vi "finalProject_interfaceLabVIEW.vi"(5 "stop":bool) -> (1 "Últimos Valores Registados:":string[](array[string]), 2 "Array":string[](array[string]), 3 "Waveform Chart":dynamicdata(graph)=[{"t0"=timestamp(3816698513.7637887 s since 1904-01-01), "dt"=1.0, "Y"=[0.0]}, {"t0"=timestamp(3816698513.7637887 s since 1904-01-01), "dt"=1.0, "Y"=[28.961962479327045]}])   [LabVIEW 2024]
uses:
  <vilib>/Instr/_visa.llb/VISA Flush IO Buffer Mask.ctl
  <vilib>/Platform/TimedLoop/XDataNode/timing_clust.ctl
  <vilib>/Platform/TimedLoop/XDataNode/nitl_modes.ctl
  <vilib>/Platform/TimedLoop/XDataNode/wakeup.ctl
  <vilib>/Utility/file.llb/Write Delimited Spreadsheet (string).vi
  <vilib>/Instr/_visa.llb/VISA Configure Serial Port (Instr).vi
  <vilib>/platform/TimedLoop/XDataNode/XDataNode.xnode
  <vilib>/Platform/TimedLoop/XDataNode/XDNodeRunTimeDep.lvlib
panel:
  out "Luminosidade (%)":sgl(slide) scale=0.0..100.0
  out "Histórico de Valores:":string[][](table)
  out "State":bool
  in  "Porta de Comunicação":refnum<visa-resource-name>="COM3-1"
  in  "Temp Setpoint (ºC)":sgl(knob)=25.0 scale=15.0..30.0 scale format="%#_2f"
  out "Temp Medida (ºC)":dbl(slide) scale=10.0..30.0
  out "Última Mensagem recebida do Arduino:":string
  in  "Diretoria de Dados Guardados:":path=path "C:/Users/celin/Documents/Alexandre Escola/Universidade/FEUP - Faculdade de Engenharia do Porto/1º Semestre/ASM - Aplicações de Sistemas Mecatrónicos/Arduino+LabView/Results.xls"
  # "Verde: Sistema Operacional\nAmarelo: Sistema Não Operacional"
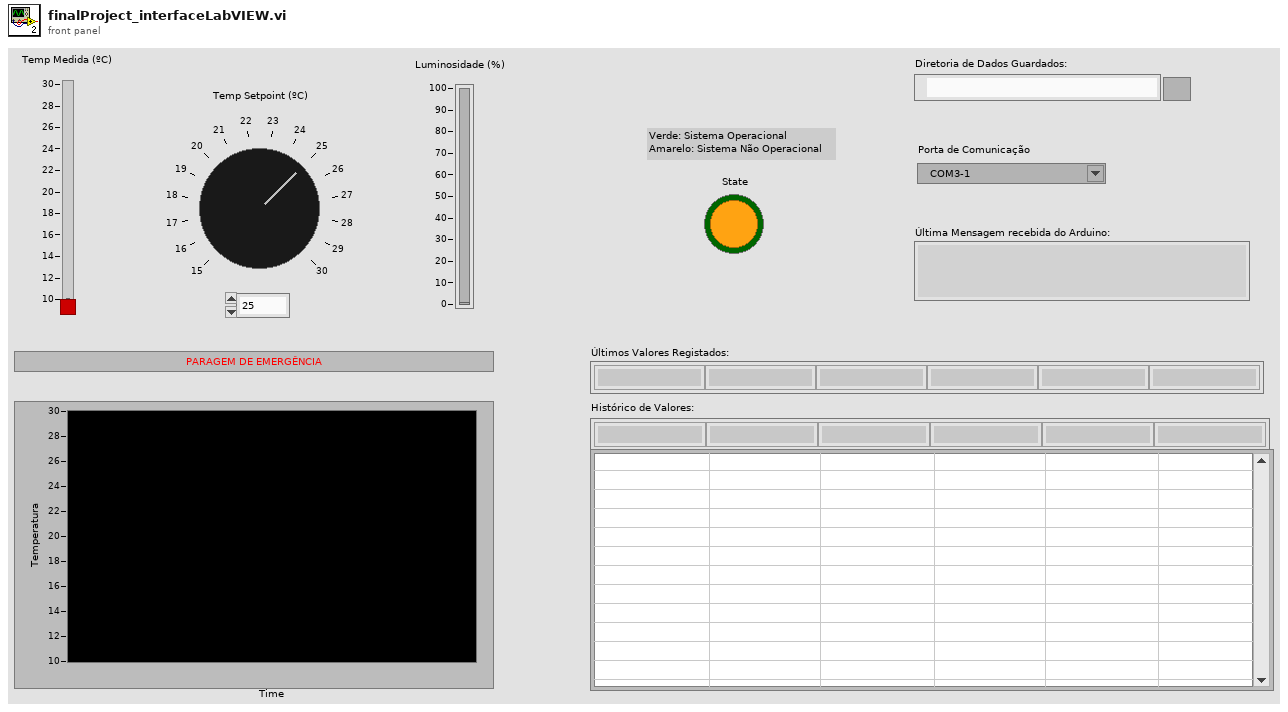
[diagram p1: front panel]
types:
  T1 = typedef "XDNodeRunTimeDep.lvlib/timing_clust.ctl" = cluster{"Expected End [f-1]":u64, "Actual End [f-1]":u64, "Finished Late? [f-1]":bool, "Expected End [i-1]":u64, "Actual End [i-1]":u64, "Finished Late? [i-1]":bool, "Expected Start [i]":u64, "Actual Start [i]":u64, "Expected Start [f]":u64, "Actual Start [f]":u64, "Source Name":string, "Structure Name":string, "Period":i64, "Deadline":i64, "Offset":i64, "Start":i64, "Priority":i32, "Timeout":i32, "Mode":T2, "Wakeup Reason":T3, "Error":errorcluster, "Source Type":string, "Secondary Source Type":string, "Global End Time":u64, "Global Start Time":u64, "Frame Duration":u64, "Iteration Duration":u64, "Assigned CPU":i32, "I/O Scan Engine Mode":u32}
  T2 = typedef "XDNodeRunTimeDep.lvlib/nitl_modes.ctl" = enum32{"No Change", "Process missed periods, maintain original phase", "Discard missed periods, maintain original phase", "Process missed periods, ignore original phase", "Discard missed periods, ignore original phase"}
  T3 = typedef "XDNodeRunTimeDep.lvlib/wakeup.ctl" = enum32{"Normal", "Aborted", "Asynchronous wakeup", "Timing source error", "Timed loop error", "Timeout"}
  T4 = typedef "VISA Flush IO Buffer Mask.ctl" = u16
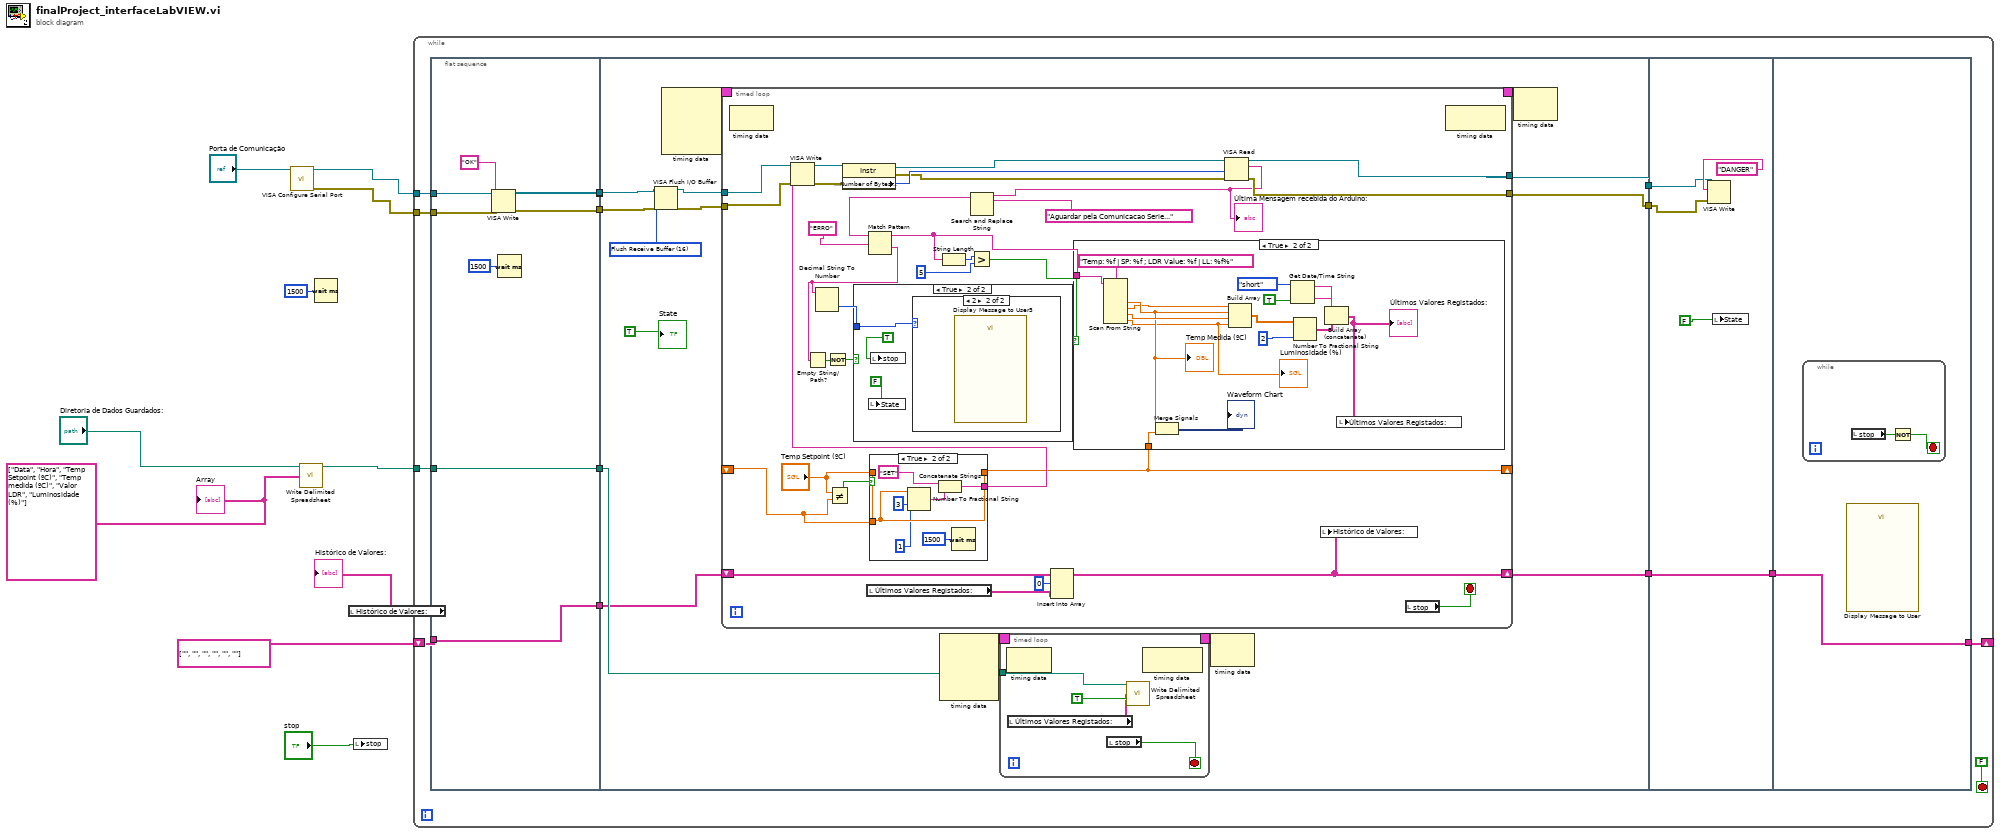
[diagram p0: block diagram]
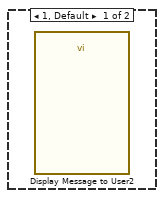
[diagram p3: hidden frame]
diagram:
  w8 = string[] ["Data", "Hora", "Temp Setpoint (ºC)", "Temp medida (ºC)", "Valor LDR", "Luminosidade (%)"]
  n1 = call-poly "VISA Configure Serial Port"("VISA resource name"="Porta de Comunicação") -> ("VISA resource name out"=w4:refnum<visa-resource-name>, "error out"=w5:errorcluster)  [unwired: 13 in]
  n2 = call-poly <vilib>:"Write Delimited Spreadsheet.vi"("file path (dialog if empty)"="Diretoria de Dados Guardados:", "1D data"=w8) -> ("new file path (Not A Path if cancelled)"=w7:path)  [unwired: 12 in, 1 out]
  n3 = Wait (ms)(milliseconds to wait=u32 1500) -> ()  [unwired: 1 out]
  n4 = local read "Histórico de Valores:"() -> (→"Histórico de Valores:":string[][])
  n5 = local write "stop"("stop") -> ()
  n6 = while {
    tunnel: w7 -> [w19]
    tunnel: w5 -> [w16]
    tunnel: w4 -> [w15]
    shift-right: [w12] -> _
    shift-left: string[][] [["", "", "", "", "", ""]] -> [w11]
    stop <- FALSE stop-if-true
    n7 = flat-sequence {
      tunnel: [w32] -> w25
      tunnel: [w31] -> w24
      tunnel: [w30] -> w23
      tunnel: [w29] -> w22
      tunnel: w15 -> [w32]
      tunnel: w16 -> [w31]
      tunnel: w19 -> [w30]
      tunnel: [w26] -> w17
      tunnel: w11 -> [w26]
      tunnel: w25 -> [_]
      tunnel: w24 -> [w35]
      tunnel: w23 -> [w41]
      tunnel: [w47] -> w21
      tunnel: [w46] -> w20
      tunnel: w22 -> [w40]
      tunnel: w17 -> [w37]
      tunnel: [w33] -> w14
      tunnel: w21 -> [w120]
      tunnel: w20 -> [w121]
      tunnel: w14 -> [w118]
      tunnel: [w118] -> w13
      tunnel: w13 -> [w123]
      tunnel: [w123] -> w12
      frame #0 {
        n8 = VISA Write(VISA resource name=w32, write buffer="OK", error in (no error)=w31) -> (VISA resource name out=w29:refnum<visa-resource-name>)  [unwired: 2 out]
        n9 = Wait (ms)(milliseconds to wait=u32 1500) -> ()  [unwired: 1 out]
      }
      frame #1 {
        w38 = T4 16 items=["Flush Receive Buffer"=16, "Write Transmit Buffer to Device"=32, "Flush Receive Buffer (No I/O)"=64, "Flush Transmit Buffer"=128] ("Mask")
        n10 = VISA Flush I/O Buffer(VISA resource name=w40, mask (16)=w38, error in (no error)=w35) -> (VISA resource name out=w39:refnum<visa-resource-name>, error out=w36:errorcluster)
        n11 = node-c288() -> (w45:T1)  [unwired: 4 in]
        n12 = timed-loop {
          tunnel: [w86] -> w46
          tunnel: [w85] -> w47
          shift-right: [w56] -> _
          shift-left: _ -> [w76]
          timing: w45 -> [_]
          timing-out: [_] -> w44
          tunnel: w39 -> [w75]
          shift-right: [w57] -> w33
          shift-left: w37 -> [w73]
          tunnel: w36 -> [w63]
          stop <- w74 stop-if-true
          n13 = node-c288() -> ()  [unwired: 1 in, 1 out]
          n14 = Not Equal?(x="Temp Setpoint (ºC)", y=w76) -> (x != y?=w78:bool)
          n15 = local read "Últimos Valores Registados:"() -> (w72:string[])
          n16 = case shown="True" w78 {
            tunnel: [w108 w113] -> w56
            tunnel: "Temp Setpoint (ºC)" -> [_ w113]
            tunnel: [_ w111] -> w81
            tunnel: w76 -> [w108 _]
            frame False {
            }
            frame True {
              n17 = Number To Fractional String(number=w113, width (-)=i16 3, precision (6)=i16 1 ("width (-)")) -> (F-format string=w114:string)  [unwired: 1 in]
              n18 = Concatenate Strings("SET", w114) -> (w111:string)
              n19 = Wait (ms)(milliseconds to wait=u32 1500) -> ()  [unwired: 1 out]
            }
          }
          n20 = VISA Write(VISA resource name=w75, write buffer=w81, error in (no error)=w63) -> (VISA resource name out=w80:refnum<visa-resource-name>, error out=w79:errorcluster)  [unwired: 1 out]
          n21 = property class="Instr"(reference=w80, error in=w79) -> (reference out=w84:refnum<visa-resource-name>, error out=w82:errorcluster, "Serial Settings:Number of Bytes at Serial Port"=w83:u32)
          n22 = Insert Into Array(array=w73, index (row)=0, new element=w72) -> (w57:string[][])  [unwired: 1 in]
          n23 = VISA Read(VISA resource name=w84, byte count=w83, error in (no error)=w82) -> (VISA resource name out=w86:refnum<visa-resource-name>, read buffer=w67:string, error out=w85:errorcluster)  [unwired: 1 out]
          "Última Mensagem recebida do Arduino:" <- w67
          n24 = Search and Replace String(input string=w67, search string="Aguardar pela Comunicacao Serie...") -> (result string=w66:string)  [unwired: 6 in, 3 out]
          n25 = Match Pattern(string=w66, regular expression="ERRO") -> (before substring=w70:string, after substring=w58:string)  [unwired: 1 in, 2 out]
          n26 = Empty String/Path?(string/path=w58) -> (empty?=w61:bool)
          n27 = Decimal String To Number(string=w58) -> (number=w59:i32)  [unwired: 2 in, 1 out]
          n28 = Not(x=w61) -> (.not. x?=w60:bool)
          n29 = case shown="True" w60 {
            tunnel: w59 -> [_ w89]
            frame False {
            }
            frame True {
              n30 = local write "State"(FALSE ("Boolean")) -> ()
              n31 = local write "stop"(TRUE ("stop")) -> ()
              n32 = case shown="2" w89 {
                frame 1, Default {
                  n33 = call "Display Message to User2"() -> ()  [unwired: 10 in, 2 out]
                }
                frame 2 {
                  n34 = call "Display Message to User3"() -> ()  [unwired: 10 in, 2 out]
                }
              }
            }
          }
          n35 = String Length(string=w70) -> (length=w69:i32)
          n36 = Greater?(x=w69, y=5) -> (0:w68:bool)
          n37 = case shown="True" w68 {
            tunnel: w70 -> [_ w93]
            tunnel: w56 -> [_ w90]
            frame False {
            }
            frame True {
              n38 = Scan From String(format string="Temp: %f | SP: %f ; LDR Value: %f | LL: %f%", input string=w93) -> (output 1=w97:dbl, output 2=w91:dbl, output 3=w104:dbl, output 4=w92:sgl)  [unwired: 6 in, 3 out]
              "Temp Medida (ºC)" <- w97
              "Luminosidade (%)" <- w92
              n39 = Merge Signals(w97, w90) -> (→"Waveform Chart":dynamicdata)
              n40 = Build Array(w91, w97, w104, w92) -> (w96:dbl[])
              n41 = Get Date/Time String(date format (0)=enum16{"short", "long", "abbreviated"}."short", want seconds? (F)=TRUE) -> (date string=w101:string, time string=w100:string)  [unwired: 1 in]
              n42 = Number To Fractional String(number=w96, precision (6)=i16 2) -> (F-format string=w102:string[])  [unwired: 2 in]
              n43 = Build Array (concatenate)(w101, w100, w102) -> (w95:string[])
              "Últimos Valores Registados:" <- w95
              n44 = local write "Últimos Valores Registados:"(w95) -> ()
            }
          }
          n45 = local write "Histórico de Valores:"(w57) -> ()
          n46 = local read "stop"() -> (w74:bool)
          n47 = node-c288() -> ()  [unwired: 1 in, 1 out]
        }
        n48 = node-c288() -> (w43:T1)  [unwired: 4 in]
        n49 = timed-loop {
          timing: w43 -> [_]
          timing-out: [_] -> w42
          tunnel: w41 -> [w51]
          stop <- w49 stop-if-true
          n50 = node-c288() -> ()  [unwired: 1 in, 1 out]
          n51 = local read "Últimos Valores Registados:"() -> (w48:string[])
          n52 = local read "stop"() -> (w49:bool)
          n53 = call-poly <vilib>:"Write Delimited Spreadsheet.vi"("file path (dialog if empty)"=w51, "1D data"=w48, "append to file? (new file:F)"=TRUE) -> ()  [unwired: 11 in, 2 out]
          n54 = node-c288() -> ()  [unwired: 1 in, 1 out]
        }
        n55 = node-c288(w42) -> ()  [unwired: 1 out]
        n56 = node-c288(w44) -> ()  [unwired: 1 out]
        "State" <- TRUE ("Boolean")
      }
      frame #2 {
        n57 = VISA Write(VISA resource name=w121, write buffer="DANGER", error in (no error)=w120) -> ()  [unwired: 3 out]
        n58 = local write "State"(FALSE) -> ()
      }
      frame #3 {
        n59 = while {
          stop <- w124 stop-if-true
          n60 = local read "stop"() -> (w125:bool)
          n61 = Not(x=w125) -> (.not. x?=w124:bool)
        }
        n62 = call "Display Message to User"() -> ()  [unwired: 10 in, 2 out]
      }
    }
  }
  "Array" <- w8
